vi "Avi_player.vi"() -> ()   [LabVIEW 2009]
panel:
  out "x-y":dbl
  out "current frame":i32
  out "time (s)":dbl
  in  "Slide":dbl(slide) max=471.7241379310345 scale=0.0..471.7241379310345 scale format="%<%H:%M:%S%3u>t"
  out "Frame Data":T1
  in  "AVI Path":path
  in  "stop":bool
  out "Number of Frames":u32
  out "Image":T2(plugin-control)
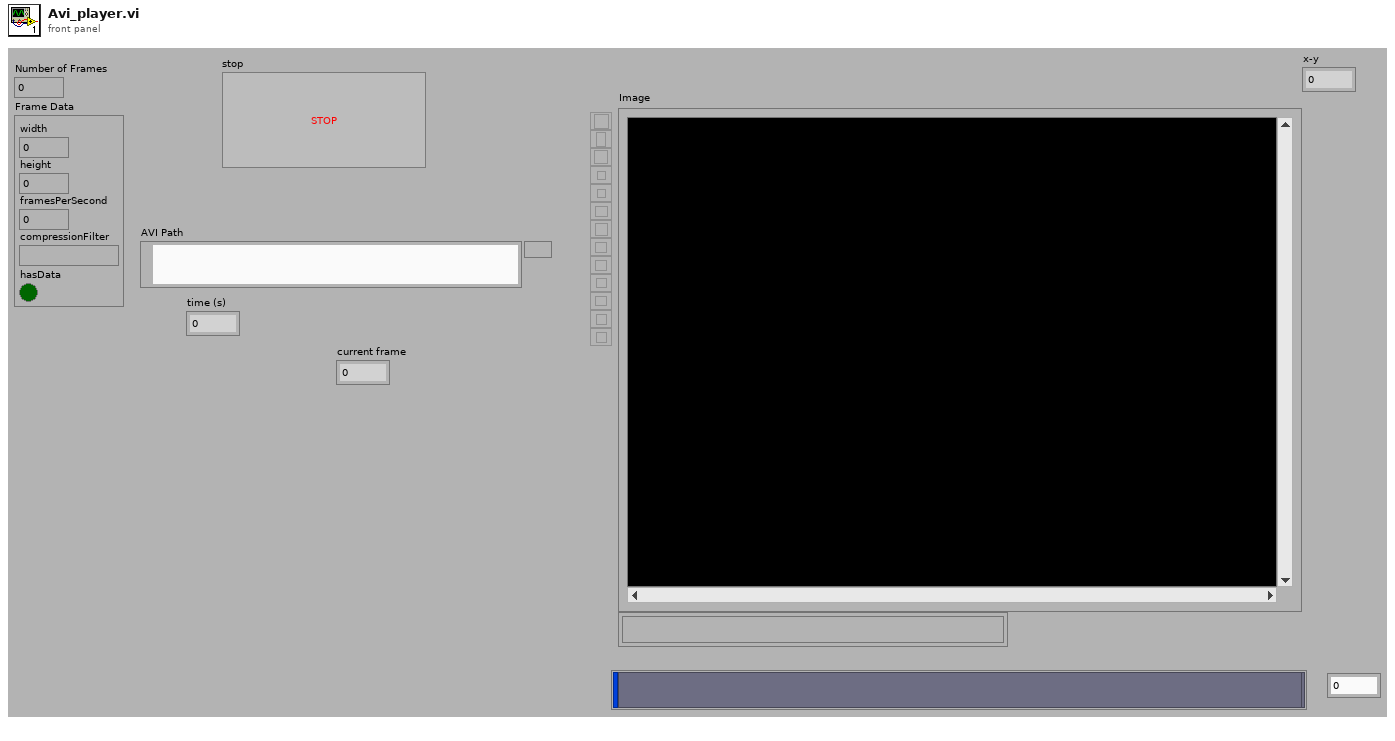
[diagram p1: front panel]
types:
  T1 = cluster{"width":u32, "height":u32, "framesPerSecond":u32, "compressionFilter":string, "hasData":bool}
  T2 = typedef "IMAQ Image.ctl" = refnum<image>
  T3 = typedef "Image Type" = u32
  T4 = typedef "AviRefnum.ctl" = refnum<k1>
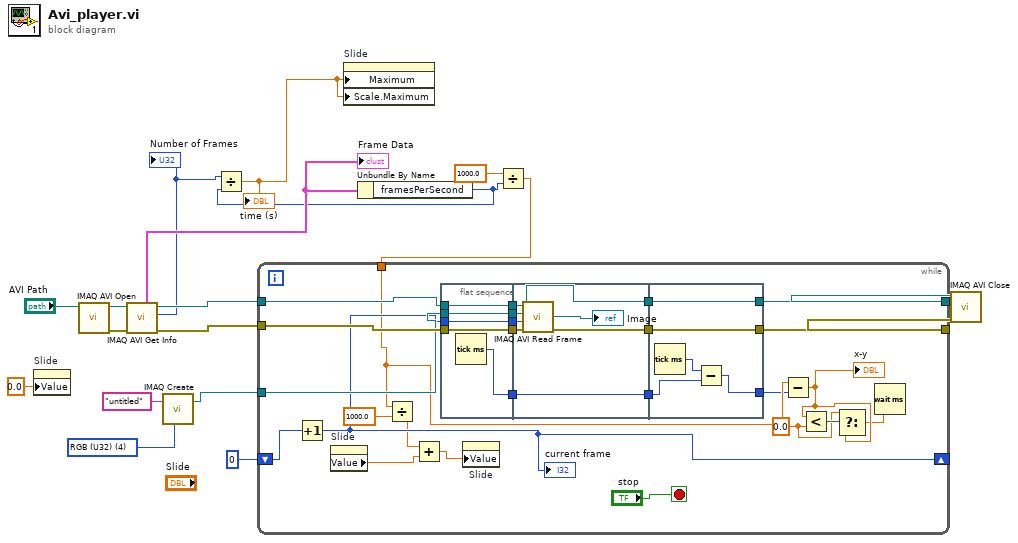
[diagram p0: block diagram]
diagram:
  w8 = T3 4 items=["Grayscale (U8)", "Grayscale (I16)", "Grayscale (SGL)", "Complex (CSG)", "RGB (U32)", "HSL (U32)", "RGB (U64)", "Grayscale (U16)"] ("Image Type")
  n1 = property on="Slide" class="Slide (strict)"("Value"=0.0 ("Slide")) -> ()  [unwired: 2 in, 2 out]
  n2 = call "IMAQ AVI Open"("AVI Path"="AVI Path") -> ("error out"=w17:errorcluster, "Avi Refnum"=w18:T4)  [unwired: 9 in]
  n3 = call "IMAQ AVI Get Info"("error in (no error)"=w17, "Avi Refnum"=w18) -> ("error out"=w14:errorcluster, "Number of Frames"=w5:u32, "Avi Refnum (duplicate)"=w16:T4, "Frame Data"=w12:T1)  [unwired: 5 in, 1 out]
  "Number of Frames" <- w5
  "Frame Data" <- w12
  n4 = call "IMAQ Create"("Image Name"="untitled", "Image Type"=w8) -> ("New Image"=w7:T2)  [unwired: 3 in, 1 out]
  n5 = Unbundle By Name(w12) -> ("framesPerSecond"=w4:u32)
  n6 = Divide(x=w5, y=w4) -> (x/y=w3:dbl)
  "time (s)" <- w3
  n7 = property on="Slide" class="Slide (strict)"("Maximum"=w3, "Scale.Maximum"=w3) -> ()  [unwired: 2 in, 2 out]
  n8 = Divide(x=1000.0, y=w4) -> (x/y=w10:dbl)
  n9 = while {
    tunnel: w16 -> [w44]
    tunnel: [w43] -> w15
    tunnel: w14 -> [w42]
    tunnel: w10 -> [w24]
    tunnel: w7 -> [w40]
    tunnel: [w39] -> w6
    shift-right: [w35] -> _
    shift-left: 0 ("current frame") -> [w38]
    stop <- "stop" stop-if-true
    w21 = 0.0 ("y")
    n10 = Increment(x=w38) -> (x+1=w35:i32)
    "current frame" <- w35
    n11 = property on="Slide" class="Slide (strict)"() -> ("Value"=w36:dbl)  [unwired: 2 in, 2 out]
    n12 = Divide(x=w24, y=1000.0) -> (x/y=w33:dbl)
    n13 = Add(x=w33, y=w36) -> (x+y=w37:dbl)
    n14 = flat-sequence {
      tunnel: w35 -> [w46]
      tunnel: w40 -> [w47]
      tunnel: w42 -> [w48]
      tunnel: w44 -> [w49]
      tunnel: [w49] -> w32
      tunnel: [w48] -> w31
      tunnel: [w47] -> w30
      tunnel: [w46] -> w29
      tunnel: [w45] -> w25
      tunnel: w32 -> [w57]
      tunnel: w31 -> [w55]
      tunnel: w30 -> [w54]
      tunnel: w29 -> [w51]
      tunnel: [w56] -> w28
      tunnel: [w52] -> w27
      tunnel: [w50] -> w26
      tunnel: w25 -> [w50]
      tunnel: [w61] -> w39
      tunnel: [w62] -> w43
      tunnel: w28 -> [w62]
      tunnel: w27 -> [w61]
      tunnel: w26 -> [w59]
      tunnel: [w58] -> w23
      frame #0 {
        n15 = Tick Count (ms)() -> (millisecond timer value=w45:u32)
      }
      frame #1 {
        n16 = call "IMAQ AVI Read Frame"("error in (no error)"=w55, "Frame Number"=w51, "Image"=w54, "Avi Refnum"=w57) -> ("error out"=w52:errorcluster, "Image Out"=→"Image":T2, "Avi Refnum (duplicate)"=w56:T4)  [unwired: 4 in, 1 out]
      }
      frame #2 {
        n17 = Tick Count (ms)() -> (millisecond timer value=w60:u32)
        n18 = Subtract(x=w60, y=w59) -> (x-y=w58:u32)
      }
    }
    n19 = property on="Slide" class="Slide (strict)"("Value"=w37) -> ()  [unwired: 2 in, 2 out]
    n20 = Subtract(x=w24, y=w23) -> (x-y=w20:dbl)
    "x-y" <- w20
    n21 = Less?(x=w20, y=w21) -> (x < y?=w22:bool)
    n22 = Select(t=w21, s=w22, f=w20) -> (s? t:f=w19:dbl)
    n23 = Wait (ms)(milliseconds to wait=w19) -> ()  [unwired: 1 out]
  }
  n24 = call "IMAQ AVI Close"("error in (no error)"=w6, "Avi Refnum"=w15) -> ()  [unwired: 9 in, 1 out]
